vi "Identify Ball.vi"(11 "Raw Image":T2) -> (2 "Ball Data":T1(array[cluster]), 3 "Ball Position":T2)   [LabVIEW 2012]
uses:
  <vilib>/vision/Image Controls.llb/IMAQ Image.ctl
  <vilib>/vision/NI_Vision_Development_Module.lvlib
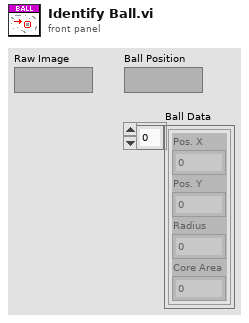
[diagram p1: front panel]
types:
  T1 = cluster{"Pos. X":i32, "Pos. Y":i32, "Radius":i32, "Core Area":i32}[]
  T2 = typedef "IMAQ Image.ctl" = refnum<image>
  T3 = enum32{"AutoM", "Close", "Dilate", "Erode", "Gradient", "Gradient in", "Gradient out", "HitMiss", "Open", "PClose", "POpen", "Thick", "Thin"}
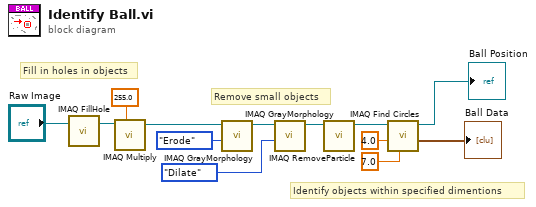
[diagram p0: block diagram]
diagram:
  # "Identify objects within specified dimentions"
  # "Remove small objects"
  # "Fill in holes in objects"
  n1 = call "IMAQ FillHole"("Image Src"="Raw Image") -> ("Image Dst Out"=w13:T2)  [unwired: 5 in, 1 out]
  n2 = call "IMAQ Multiply"("Image Src A"=w13, "Constant"=sgl 255.0) -> ("Image Dst Out"=w2:T2)  [unwired: 5 in, 1 out]
  n3 = call "IMAQ GrayMorphology"("Operation"=T3."Erode", "Image Src"=w2) -> ("Image Dst Out"=w5:T2)  [unwired: 8 in, 1 out]
  n4 = call "IMAQ GrayMorphology"("Operation"=T3."Dilate", "Image Src"=w5) -> ("Image Dst Out"=w10:T2)  [unwired: 8 in, 1 out]
  n5 = call "IMAQ RemoveParticle"("Image Src"=w10) -> ("Image Dst Out"=w9:T2)  [unwired: 9 in, 1 out]
  n6 = call "IMAQ Find Circles"("Max Radius"=sgl 7.0, "Min Radius"=sgl 4.0, "Image Src"=w9) -> ("Circles Data"=→"Ball Data":T1, "Image Dst Out"=→"Ball Position":T2)  [unwired: 5 in, 2 out]
